vi "VI Tree - array__ogtk.vi"   [LabVIEW 2019]
uses:
  Sort 2D Array (DBL)__ogtk.vi
  Reverse 2D Array (SGL)__ogtk.vi
  Empty 1D Array (DBL)__ogtk.vi
  Slice 1D Array (DBL)__ogtk.vi
  Remove Duplicates from 1D Array (DBL)__ogtk.vi
  Filter 1D Array (DBL)__ogtk.vi
  Conditional Auto-Indexing Tunnel (DBL)__ogtk.vi
  Search 1D Array (DBL)__ogtk.vi
  Sort 1D Array (DBL)__ogtk.vi
  Index 1D Array Elements (DBL)__ogtk.vi
  Delete Elements from 1D Array (DBL)__ogtk.vi
  Reorder 2D Array (DBL)__ogtk.vi
  Reorder 2D Array2 (DBL)__ogtk.vi
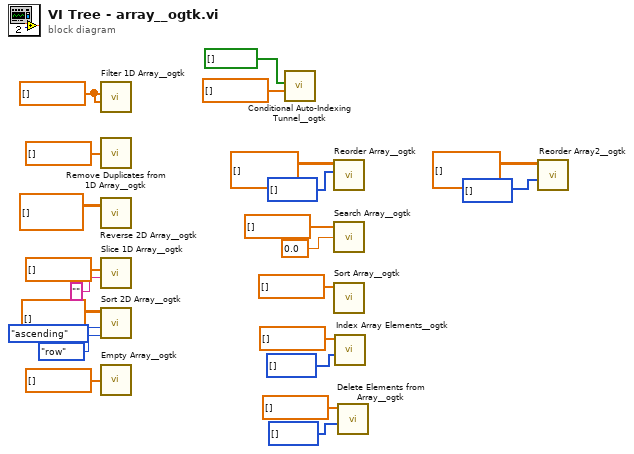
[diagram p0: block diagram]
diagram:
  w21 = dbl[] [] ("Array")
  n1 = call-poly "Filter 1D Array__ogtk.vi"("items to filter"=w21, "array"=w21) -> ()  [unwired: 4 in, 2 out]
  n2 = call-poly "Remove Duplicates from 1D Array__ogtk.vi"("Input Array"=dbl[] []) -> ()  [unwired: 2 out]
  n3 = call-poly "Reverse 2D Array__ogtk.vi"("Array"=sgl[][] []) -> ()  [unwired: 2 in, 1 out]
  n4 = call-poly "Slice 1D Array__ogtk.vi"("slice"="", "array"=dbl[] []) -> ()  [unwired: 5 in, 1 out]
  n5 = call-poly "Sort 2D Array__ogtk.vi"("Sort By in"=enum16{"row", "column"}."row", "Order"=enum16{"ascending", "descending"}."ascending", "Array in"=dbl[][] []) -> ()  [unwired: 5 in, 4 out]
  n6 = call-poly "Empty Array__ogtk.vi"("Array"=dbl[] []) -> ()  [unwired: 8 in, 1 out]
  n7 = call-poly "Conditional Auto-Indexing Tunnel__ogtk.vi"("Array in"=dbl[] [], "Elements to keep"=bool[] []) -> ()  [unwired: 5 in, 1 out]
  n8 = call-poly "Reorder Array__ogtk.vi"("Sorted Pointers in"=i32[] [], "Array in"=dbl[][] []) -> ()  [unwired: 7 in, 3 out]
  n9 = call-poly "Search Array__ogtk.vi"("Array"=dbl[] [], "Element Data"=0.0) -> ()  [unwired: 7 in, 1 out]
  n10 = call-poly "Sort Array__ogtk.vi"("Array in"=dbl[] []) -> ()  [unwired: 9 in, 2 out]
  n11 = call-poly "Index Array Elements__ogtk.vi"("indices"=i32[] [], "array"=dbl[] []) -> ()  [unwired: 9 in, 1 out]
  n12 = call-poly "Delete Elements from Array__ogtk.vi"("indices"=i32[] [], "array"=dbl[] []) -> ()  [unwired: 8 in, 2 out]
  n13 = call-poly "Reorder Array2__ogtk.vi"("indices"=i32[] [] ("Sorted Pointers in"), "array"=dbl[][] [] ("Array in")) -> ()  [unwired: 9 in, 1 out]
